vi "CSConnectGUI.mergeStatus.vi"(1 "Input1":i32, 4 "Input2":i32) -> (15 "Out":i32)   [LabVIEW 2014, in "CSConnectGUI.lvlib"]
doc: "Calculates a common status for the InChannel."
uses:
  CSConnectGUI.lvlib
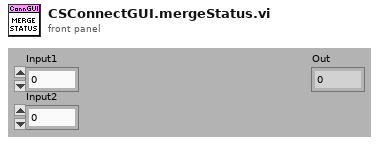
[diagram p1: front panel]
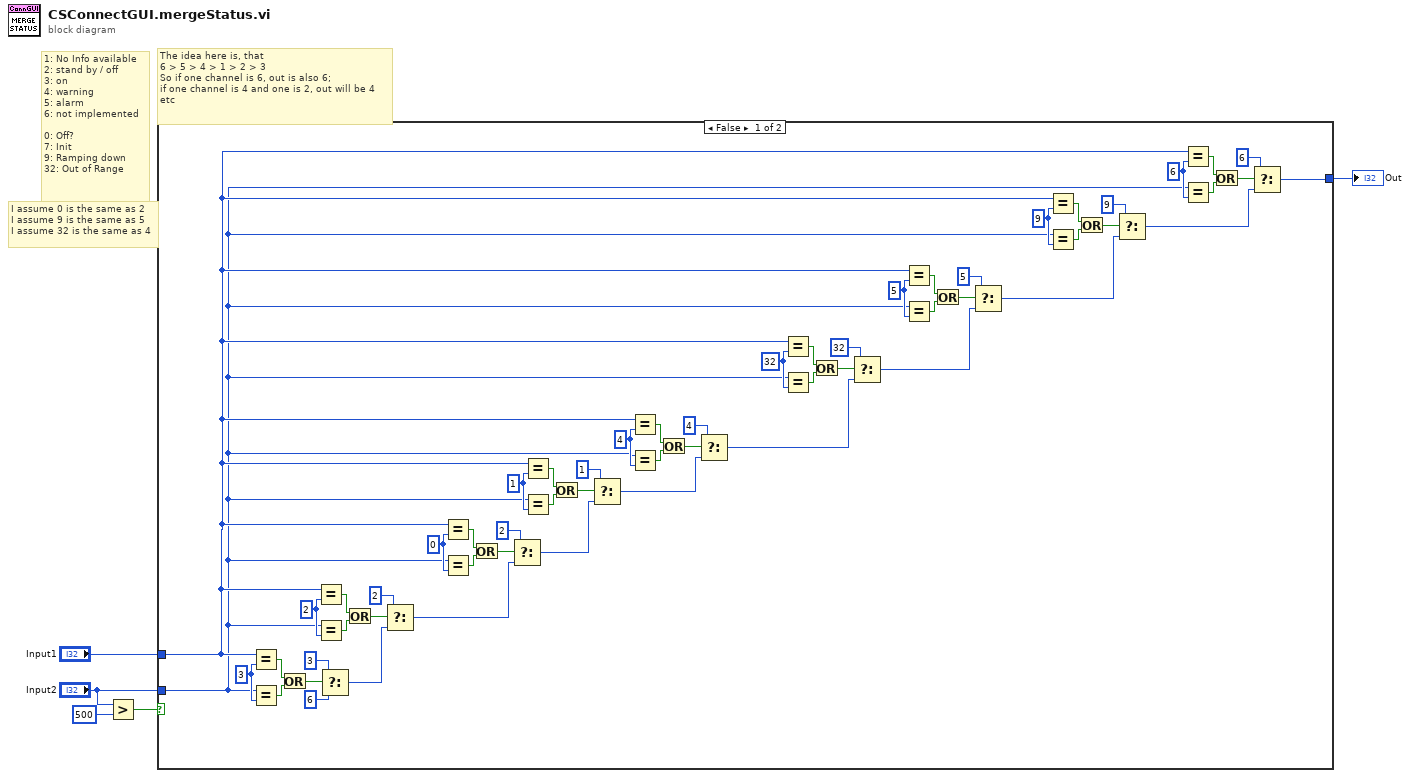
[diagram p0: block diagram]
diagram:
  # "I assume 0 is the same as 2\nI assume 9 is the same as 5\nI assume 32 is the same as 4"
  # "The idea here is, that \n6 > 5 > 4 > 1 > 2 > 3\nSo if one channel is 6, out is also 6;\nif one channel is 4 and one is 2, out will be 4\netc"
  # "1: No Info available\n2: stand by / off\n3: on\n4: warning\n5: alarm\n6: not implemented\n\n0: Off?\n7: Init\n9: Ramping down\n32: Out of Range"
  n1 = Greater?(x="Input2", y=500) -> (0:w1:bool)
  n2 = case shown="False" w1 {
    tunnel: "Input1" -> [w9 w63]
    tunnel: "Input2" -> [w8 _]
    tunnel: [w29 w63] -> w4
    frame False {
      w10 = 32 ("y")
      w17 = 9 ("y")
      w24 = 0 ("y")
      w31 = 6 ("y")
      w36 = 5 ("y")
      w42 = 4 ("y")
      w47 = 1 ("y")
      w53 = 2 ("y")
      w58 = 3 ("y")
      n3 = Equal?(x=w9, y=w58) -> (x = y?=w59:bool)
      n4 = Equal?(x=w8, y=w58) -> (x = y?=w60:bool)
      n5 = Or(x=w59, y=w60) -> (x .or. y?=w61:bool)
      n6 = Equal?(x=w9, y=w53) -> (x = y?=w54:bool)
      n7 = Equal?(x=w8, y=w53) -> (x = y?=w55:bool)
      n8 = Select(t=3 ("y"), s=w61, f=6 ("y")) -> (s? t:f=w52:i32)
      n9 = Or(x=w54, y=w55) -> (x .or. y?=w56:bool)
      n10 = Select(t=2 ("y"), s=w56, f=w52) -> (s? t:f=w22:i32)
      n11 = Equal?(x=w9, y=w24) -> (x = y?=w25:bool)
      n12 = Equal?(x=w8, y=w24) -> (x = y?=w26:bool)
      n13 = Or(x=w25, y=w26) -> (x .or. y?=w27:bool)
      n14 = Select(t=2 ("y"), s=w27, f=w22) -> (s? t:f=w23:i32)
      n15 = Equal?(x=w9, y=w47) -> (x = y?=w48:bool)
      n16 = Equal?(x=w8, y=w47) -> (x = y?=w49:bool)
      n17 = Or(x=w48, y=w49) -> (x .or. y?=w50:bool)
      n18 = Select(t=1 ("y"), s=w50, f=w23) -> (s? t:f=w41:i32)
      n19 = Equal?(x=w9, y=w42) -> (x = y?=w43:bool)
      n20 = Equal?(x=w8, y=w42) -> (x = y?=w44:bool)
      n21 = Or(x=w43, y=w44) -> (x .or. y?=w45:bool)
      n22 = Select(t=4 ("y"), s=w45, f=w41) -> (s? t:f=w7:i32)
      n23 = Equal?(x=w9, y=w10) -> (x = y?=w11:bool)
      n24 = Equal?(x=w8, y=w10) -> (x = y?=w12:bool)
      n25 = Or(x=w11, y=w12) -> (x .or. y?=w13:bool)
      n26 = Select(t=32 ("y"), s=w13, f=w7) -> (s? t:f=w6:i32)
      n27 = Equal?(x=w9, y=w36) -> (x = y?=w37:bool)
      n28 = Equal?(x=w8, y=w36) -> (x = y?=w38:bool)
      n29 = Or(x=w37, y=w38) -> (x .or. y?=w39:bool)
      n30 = Select(t=5 ("y"), s=w39, f=w6) -> (s? t:f=w16:i32)
      n31 = Equal?(x=w9, y=w17) -> (x = y?=w18:bool)
      n32 = Equal?(x=w8, y=w17) -> (x = y?=w19:bool)
      n33 = Or(x=w18, y=w19) -> (x .or. y?=w20:bool)
      n34 = Select(t=9 ("y"), s=w20, f=w16) -> (s? t:f=w15:i32)
      n35 = Equal?(x=w9, y=w31) -> (x = y?=w32:bool)
      n36 = Equal?(x=w8, y=w31) -> (x = y?=w33:bool)
      n37 = Or(x=w32, y=w33) -> (x .or. y?=w34:bool)
      n38 = Select(t=6 ("y"), s=w34, f=w15) -> (s? t:f=w29:i32)
    }
    frame True {
    }
  }
  "Out" <- w4
